vi "Sequence State.vi"(4 "y":string) -> (1 "result":bool)   [LabVIEW 2022 SP3]
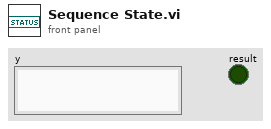
[diagram p1: front panel]
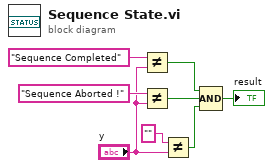
[diagram p0: block diagram]
diagram:
  n1 = Not Equal?(x="Sequence Completed", y="y") -> (x != y?=w4:bool)
  n2 = Not Equal?(x="Sequence Aborted !", y="y") -> (x != y?=w3:bool)
  n3 = Not Equal?(x="", y="y") -> (x != y?=w2:bool)
  n4 = Compound Arithmetic op=AND(w4, w3, w2) -> (→"result":bool)
